vi "Get Stack ID.vi"(8 "error in (no error)":errorcluster, 10 "Device UID":string, 11 "IP Connection in":refnum<class "IP Connection.lvclass">) -> (0 "error out":errorcluster, 1 "Sucessful":bool, 2 "Get Stack ID Response":T1, 3 "IP Connection out":refnum<class "IP Connection.lvclass">, 4 "timed out":bool)   [LabVIEW 2011, in "Tinkerforge.lvlib" / "IP Connection.lvclass"]
doc: "This VI returns the meta data of the device with the given <B>Device UID</B>."
uses:
  IP Connection.lvclass
  Type Definitions/Get Stack ID Response.ctl
  Device/Type Definitions/Firmware Version.ctl
  Type Definitions/Functions.ctl
  IP Connection.lvclass/IP Connection.ctl
  Device/Device.lvclass
  Tinkerforge.lvlib
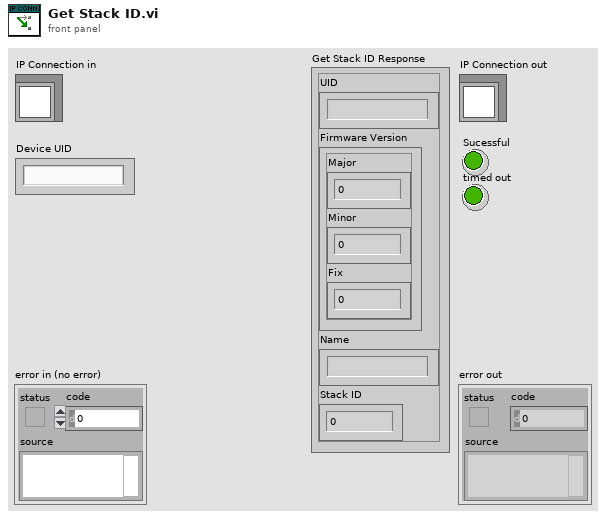
[diagram p1: front panel]
types:
  T1 = typedef "Tinkerforge.lvlib/IP Connection.lvclass/Get Stack ID Response.ctl" = cluster{"UID":string, "Firmware Version":T2, "Name":string, "Stack ID":u8}
  T2 = typedef "Tinkerforge.lvlib/Device.lvclass/Firmware Version.ctl" = cluster{"Major":u8, "Minor":u8, "Fix":u8}
  T3 = typedef "Tinkerforge.lvlib/IP Connection.lvclass/Functions.ctl" = enum8{"no Global Function", "get stack id", "enumerate", "CB enumerate"}
  T4 = enum16{"big-endian, network order", "native, host order", "little-endian"}
  T5 = typedef "Tinkerforge.lvlib/IP Connection.lvclass/Answer.ctl" = cluster{"Request GUID":string, "Request Type":T6, "Sucessful":bool, "Data":variant, "Error":errorcluster}
  T6 = typedef "Tinkerforge.lvlib/IP Connection.lvclass/Request Type.ctl" = enum8{"Invalid", "Write"}
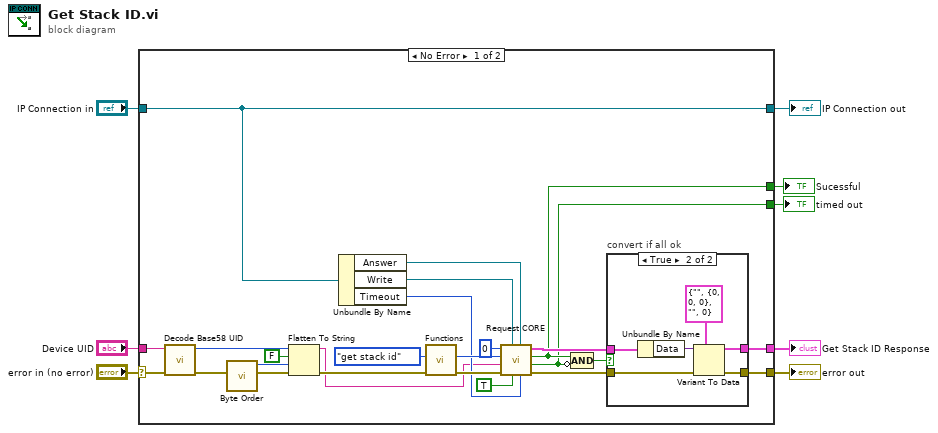
[diagram p0: block diagram]
diagram:
  n1 = case shown="No Error" "error in (no error)" {
    selector: "error in (no error)" -> [w12 w41]
    tunnel: [w17 w41] -> w7
    tunnel: [w30 w40] -> w5
    tunnel: "IP Connection in" -> [w30 w40]
    tunnel: "Device UID" -> [w9 _]
    tunnel: [w16 _] -> w3
    tunnel: [w15 _] -> w2
    tunnel: [w14 _] -> w1
    frame No Error {
      n2 = call "Decode Base58 UID.vi"("Error In"=w12, "Base58 UID"=w9) -> ("Error Out"=w11:errorcluster, "UID"=w10:u64)  [unwired: 8 in]
      n3 = call "Byte Order.vi"() -> ("byte order (2:little-endian)"=w19:T4)  [unwired: 11 in]
      n4 = Flatten To String(anything=w10, prepend array or string size? (T)=FALSE, byte order (0:big-endian, network order)=w19, error in (no error)=w11) -> (data string=w21:string, error out=w22:errorcluster)  [unwired: 1 out]
      n5 = Unbundle By Name(w30) -> ("Answer"=w29:refnum<user-event>, "Write"=w28:refnum<queue>, "Timeout"=w25:i32)
      n6 = call "Functions.vi"("Error In"=w22, "Function in"=Functions."get stack id") -> ("Error Out"=w31:errorcluster, "Function ID out"=w26:u8)  [unwired: 7 in, 1 out]
      n7 = call "Request CORE.vi"("Timeout"=w25, "Answer UE"=w29, "Response"=TRUE, "Write"=w28, "Error In"=w31, "Data"=w21, "Function ID"=w26, "Stack ID"=u8 0) -> ("Error Out"=w18:errorcluster, "timed out"=w14:bool, "Sucessful"=w15:bool, "Answer"=w23:T5)
      n8 = Compound Arithmetic op=AND(w15, invert w14) -> (w13:bool)
      n9 = case "convert if all ok" shown="True" w13 {
        tunnel: w23 -> [_ w39]
        tunnel: w18 -> [w33 w37]
        tunnel: [w33 w36] -> w17
        tunnel: [_ w34] -> w16
        frame False {
        }
        frame True {
          n10 = Unbundle By Name(w39) -> ("Data"=w38:variant)
          n11 = Variant To Data(error in=w37, type=T1 {"UID"="", "Firmware Version"={"Major"=0, "Minor"=0, "Fix"=0}, "Name"="", "Stack ID"=0} ("Get Stack ID Response"), Variant=w38) -> (data=w34:T1, error out=w36:errorcluster)
        }
      }
    }
    frame Error {
    }
  }
  "error out" <- w7
  "IP Connection out" <- w5
  "Get Stack ID Response" <- w3
  "Sucessful" <- w2
  "timed out" <- w1
